vi "subvi ACT ENC.vi"() -> (3 "Numeric":sgl)   [LabVIEW 2019]
uses:
  <vilib>/rvi/eio/common/nirviEmuTemplateMethod_errors.vi
  <vilib>/eio/EIONode/EIONode.xnode
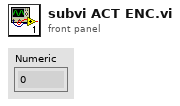
[diagram p1: front panel]
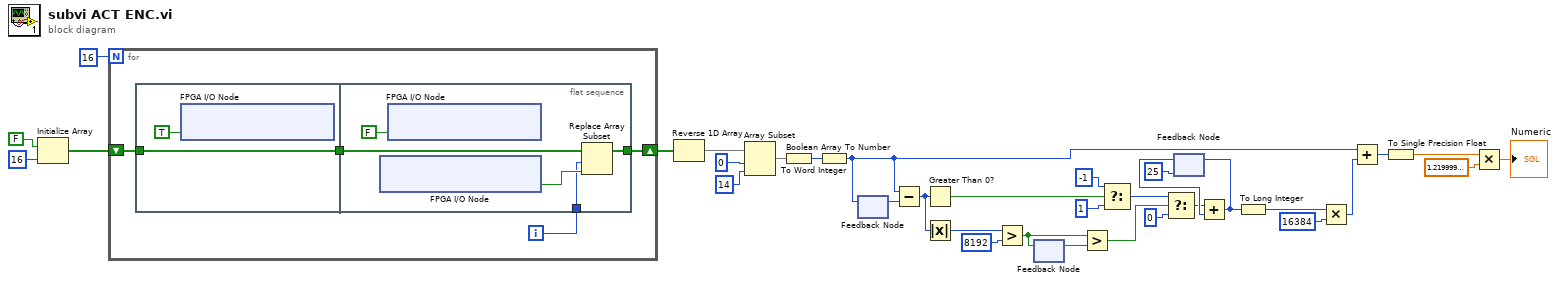
[diagram p0: block diagram]
diagram:
  n1 = Initialize Array(FALSE, 16 ("dimension size")) -> (w6:bool[])
  n2 = for {
    N: 16 -> [_]
    shift-right: [w35] -> w1
    shift-left: w6 -> [w36]
    i -> [w38]
    n3 = flat-sequence {
      tunnel: [w39] -> w37
      tunnel: w36 -> [w39]
      tunnel: w38 -> [w43]
      tunnel: w37 -> [w42]
      tunnel: [w41] -> w35
      frame #0 {
        n4 = xnode "FPGA I/O Node"("ACTUATOR ENC CLK"=TRUE ("SPI.CLK")) -> ()  [unwired: 1 in, 1 out]
      }
      frame #1 {
        n5 = xnode "FPGA I/O Node"() -> ("ACTUATOR ENC MISO"=w44:bool)  [unwired: 1 in, 1 out]
        n6 = xnode "FPGA I/O Node"("ACTUATOR ENC CLK"=FALSE ("SPI.CLK")) -> ()  [unwired: 1 in, 1 out]
        n7 = Replace Array Subset(array=w42, new element=w44, index=w43) -> (w41:bool[])
      }
    }
  }
  n8 = Reverse 1D Array(array=w1) -> (reversed array=w3:bool[])
  n9 = Array Subset(array=w3, index=0, length=14) -> (w2:bool[])
  n10 = Boolean Array To Number(Boolean array=w2) -> (number=w31:u16)
  n11 = To Word Integer(number=w31) -> (16bit integer=w25:i16)
  n12 = feedback #1() -> (w10:i16)  [unwired: 1 in]
  n13 = feedback-in #1(w25) -> ()
  n14 = Subtract(x=w25, y=w10) -> (x-y=w12:i16)
  n15 = Greater Than 0?(x=w12) -> (x > 0?=w13:bool)
  n16 = Absolute Value(x=w12) -> (abs(x)=w11:i16)
  n17 = Greater?(x=w11, y=i16 8192) -> (0:w18:bool)
  n18 = feedback #2() -> (w17:bool)  [unwired: 1 in]
  n19 = feedback-in #2(w18) -> ()
  n20 = Greater?(x=w18, y=w17) -> (0:w19:bool)
  n21 = Select(t=i16 -1, s=w13, f=i16 1) -> (s? t:f=w14:i16)
  n22 = Select(t=w14, s=w19, f=i16 0) -> (s? t:f=w15:i16)
  n23 = feedback #3(i16 25) -> (w24:i16)
  n24 = Add(x=w15, y=w24) -> (x+y=w26:i16)
  n25 = feedback-in #3(w26) -> ()
  n26 = To Long Integer(number=w26) -> (32bit integer=w27:i32)
  n27 = Multiply(x=w27, y=16384) -> (x*y=w16:i32)
  n28 = Add(x=w25, y=w16) -> (x+y=w32:i32)
  n29 = To Single Precision Float(number=w32) -> (single precision float=w33:sgl)
  n30 = Multiply(x=w33, y=sgl 1.22e-06) -> (x*y=→"Numeric":sgl)
